vi "Thev-Initialize Calibration Procedure.vi"(0 "State in":T1, 5 "Params":T5 {"LProbe" items=["None"=-1, "Probe A"=0, "Probe B"=1]; "Rprobe" items=["None"=-1, "Probe A"=0, "Probe B"=1]}) -> (4 "State out":T1, 15 "error out":errorcluster)   [LabVIEW 2015]
uses:
  Typedefs/Thev-Parameters.ctl
  Typedefs/Thev-Stimulus.ctl
  Typedefs/Thev-Find.ctl
  Misc VIs/Equipment Control/ER10X/ER10X-Probe.ctl
  Typedefs/Thev-Optimization Parameters.ctl
  Typedefs/Thev-State.ctl
  D:/Experiment VIs/Misc VIs/Equipment Control/ER10X/ER10XConnect.NET.dll
  Misc VIs/Equipment Control/ER10X/ER10XConnect.NET.dll
  Typedefs/Thev-Procedure Phase.ctl
  Typedefs/Thev-Progress Table Element.ctl
  Typedefs/Thev-Optimization Result.ctl
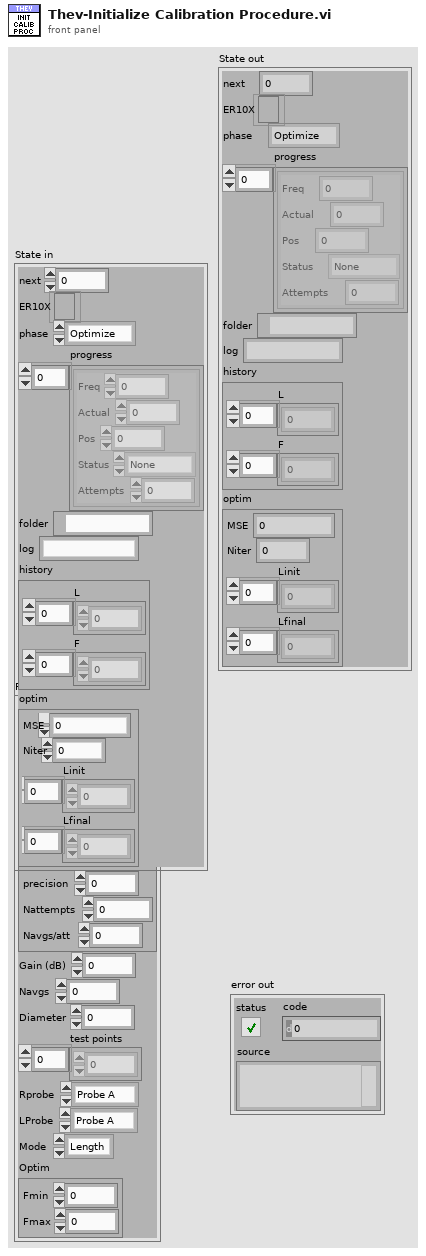
[diagram p1: front panel]
types:
  T1 = typedef "Thev-State.ctl" = cluster{"next":i32, "ER10X":refnum<k24>, "phase":T2, "progress":T3[], "folder":path, "log":string, "history":cluster{"L":dbl[], "F":dbl[]}, "optim":T4}
  T2 = typedef "Thev-Procedure Phase.ctl" = enum16{"Optimize", "Measure", "Compute", "Finished"}
  T3 = typedef "Thev-Progress Table Element.ctl" = cluster{"Freq":dbl, "Actual":dbl, "Pos":dbl, "Status":enum16{"None", "Measuring", "Finished"}, "Attempts":i32}
  T4 = typedef "Thev-Optimization Result.ctl" = cluster{"MSE":dbl, "Niter":i32, "Linit":dbl[], "Lfinal":dbl[]}
  T5 = typedef "Thev-Parameters.ctl" = cluster{"Speaker":enum16{"Right primary", "Right secondary", "Left primary", "Left secondary"}, "Chirp":T6, "Find":T7, "Gain (dB)":dbl, "Navgs":i32, "Diameter":dbl, "test points":dbl[], "Rprobe":T8, "LProbe":T8, "Mode":enum16{"Length", "Freq"}, "Optim":T9}
  T6 = typedef "Thev-Stimulus.ctl" = cluster{"resol (Hz)":dbl, "atten (dB)":dbl, "Fs (Hz)":dbl}
  T7 = typedef "Thev-Find.ctl" = cluster{"precision":dbl, "Nattempts":i32, "Navgs/att":i32}
  T8 = typedef "ER10X-Probe.ctl" = i32
  T9 = typedef "Thev-Optimization Parameters.ctl" = cluster{"Fmin":dbl, "Fmax":dbl}
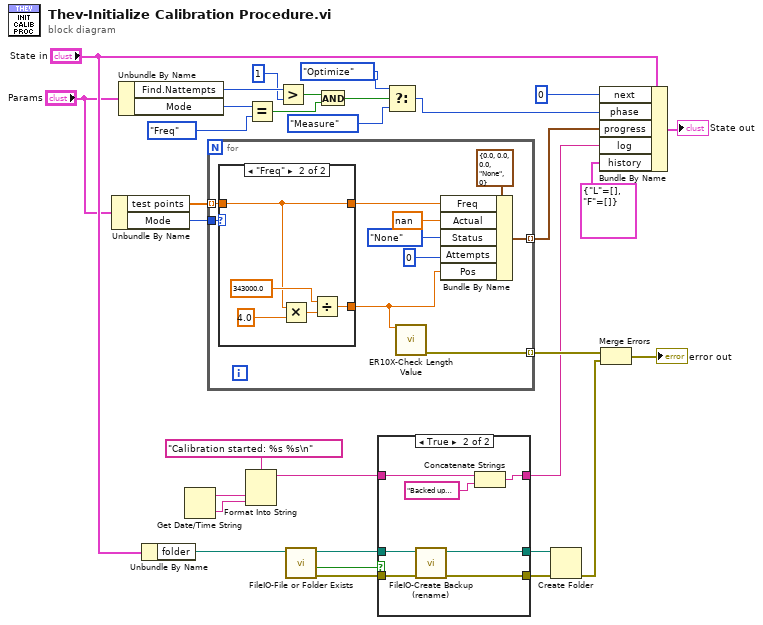
[diagram p0: block diagram]
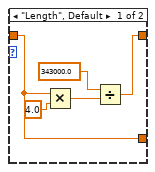
[diagram p3: hidden frame]
diagram:
  n1 = Unbundle By Name("Params") -> ("test points"=w30:dbl[], "Mode"=w1:enum16{"Length", "Freq"})
  n2 = Unbundle By Name("Params") -> ("Find.Nattempts"=w9:i32, "Mode"=w11:enum16{"Length", "Freq"})
  n3 = Unbundle By Name("State in") -> ("folder"=w13:path)
  n4 = Get Date/Time String() -> (date string=w25:string, time string=w24:string)  [unwired: 3 in]
  n5 = for {
    tunnel: w30 -> [w39] mode=indexing
    tunnel: [w41] -> w29 mode=indexing
    tunnel: [w36] -> w28 mode=indexing
    tunnel: w1 -> [w34]
    n6 = case shown="\"Freq\"" w34 {
      tunnel: w39 -> [w47 w48]
      tunnel: [w47 w49] -> w37
      tunnel: [w44 w48] -> w33
      frame "Length", Default {
        n7 = Multiply(x=w47, y=4.0) -> (x*y=w45:dbl)
        n8 = Divide(x=343000.0, y=w45) -> (x/y=w44:dbl)
      }
      frame "Freq" {
        n9 = Multiply(x=w48, y=4.0) -> (x*y=w51:dbl)
        n10 = Divide(x=343000.0, y=w51) -> (x/y=w49:dbl)
      }
    }
    n11 = call "ER10X-Check Length Value.vi"("Length (mm)"=w37) -> ("error out"=w36:errorcluster)  [unwired: 14 in]
    n12 = Bundle By Name(cluster=T3 {"Freq"=0.0, "Actual"=0.0, "Pos"=0.0, "Status"=enum."None", "Attempts"=0} ("Element"), "Freq"=w33, "Actual"=nan, "Status"=enum16{"None", "Measuring", "Finished"}."None", "Attempts"=0, "Pos"=w37) -> (w41:T3)
  }
  n13 = Format Into String(format string="Calibration started: %s %s\n", w25, w24) -> (resulting string=w23:string)  [unwired: 2 in, 1 out]
  n14 = Equal?(x=w11, y=enum16{"Length", "Freq"}."Freq") -> (x = y?=w6:bool)
  n15 = Greater?(x=w9, y=1) -> (0:w7:bool)
  n16 = call "FileIO-File or Folder Exists.vi"("path"=w13) -> ("error out"=w20:errorcluster, "Exists?"=w22:bool, "dup path"=w21:path)  [unwired: 7 in, 1 out]
  n17 = And(x=w7, y=w6) -> (x .and. y?=w5:bool)
  n18 = case shown="True" w22 {
    tunnel: w23 -> [w53 w62]
    tunnel: w21 -> [w55 w59]
    tunnel: [w55 w58] -> w19
    tunnel: w20 -> [w54 w57]
    tunnel: [w54 w56] -> w18
    tunnel: [w53 w61] -> w16
    frame False {
    }
    frame True {
      n19 = call "FileIO-Create Backup (rename).vi"("error in (no error)"=w57, "Path"=w59) -> ("error out"=w56:errorcluster, "Path (thru)"=w58:path)  [unwired: 6 in, 2 out]
      n20 = Concatenate Strings(w62, "Backed up previous calibration folder.\n" ("string")) -> (w61:string)
    }
  }
  n21 = Select(t=Thev-Procedure_Phase."Optimize" ("phase"), s=w5, f=Thev-Procedure_Phase."Measure") -> (s? t:f=w3:T2)
  n22 = Create Folder(path (use dialog)=w19, error in=w18) -> (error out=w17:errorcluster)  [unwired: 1 in, 2 out]
  n23 = Bundle By Name(cluster="State in", "next"=0, "phase"=w3, "progress"=w29, "log"=w16, "history"=cluster{"L":dbl[], "F":dbl[]} {"L"=[], "F"=[]}) -> (→"State out":T1)
  n24 = Merge Errors(w28, w17) -> (→"error out":errorcluster)
